vi "OE2012&OE2022_Configure Input Filter.vi"(7 "OE2012&OE2022_\nConfigure Input Filter":T1={"Input Source"=0, "Input Shield Grounding "=0, "Input Coupling "=0, "Input Range"=0, "Signal In Channel"=1} {"Signal In Channel" items=["Signal In 1"=1, "Signal In 2"=2]; "Input Range" items=["5V", "1V", "200mV", "50mV", "10mV", "2mV", "1mV"]; "Input Coupling" items=["AC", "DC"]; "Input Shield Grounding" items=["Float", "Ground"]; "Input Source" items=["A", "A-B", "Current"]}, 8 "Error in (no error)":errorcluster caption="error out（no error）", 9 "Remote Mode":u16(ring) items=["USB", "RS232", "GPIB", "Ethernet"], 10 "Connection ID in":refnum<k5>, 11 "VISA resource name":refnum<visa-resource-name>) -> (0 "Error out":errorcluster caption="error out", 1 "Output String":string, 2 "Connection ID out":refnum<k5>, 3 "VISA resource  out":refnum<visa-resource-name>)   [LabVIEW 2011]
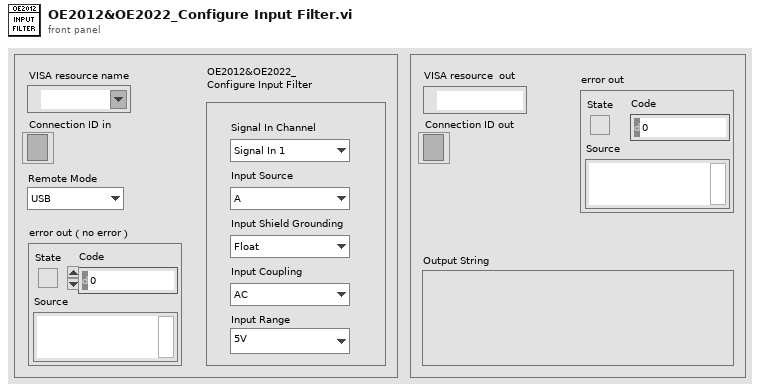
[diagram p1: front panel]
types:
  T1 = cluster{"Input Source":u16, "Input Shield Grounding ":u16, "Input Coupling ":u16, "Input Range":u16, "Signal In Channel":u16}
  T2 = enum16{"ISRC", "IGND", "ICPL", "ILIN", "PHAS", "FMOD", "RSLP", "FREQ", "SWPT", "SLLM", "SULM", "SSLL", "SSLG", "STLM", "SWRM", "IRNG", "SENS", "RMOD", "OFLT", "OFSL", "SYNC", "DMOD", "HARM", "DARB", "SWVT", "SLVL", "SVLL", "SVUL", "SVSL", "SVSG", "SVTM", "SVRM", "RALL", "SNAP", "OUTP", "OAUX", "COUT", "CAUX", "COFP", "CEXP", "FPOP", "OEXP", "*IDN", "*RST", "OVLD", "INOV", "GNOV", "*PLL", "SSET", "RSET", "AGAN", "APHS", "ARSV", "ASCL", "EQCD", "EQCS", "SPED", "SRAT", "SLEN", "SSLE", "STRG", "SPRM", "STRD", "PAUS", "REST", "SPTS", "TRCA", "TEMP", "RSTU", "IHNZ", "DEQU", "SADD", "ARNG", "CSPE", "ISRCD", "IGNDD", "ICPLD", "ILIND", "PHASD", "FMODD", "RSLPD", "FREQD", "SWPTD", "SLLMD", "SULMD", "SSLLD", "SSLGD", "STLMD", "SWRMD", "SENSD", "RMODD", "OFLTD", "OFSLD", "SYNCD", "HARMD", "EQCDD", "EQCSD", "SNAPD", "OUTPD", "SWVTD", "SLVLD", "SVLLD", "SVULD", "SVSLD", "SVSGD", "SVTMD", "SVRMD", "SVDCD", "ARSVD", "AGAND", "APHSD", "ASCLD", "FPOPD", "CAUXD", "OEXPD", "SPEDD", "SRATD", "SLEND", "SSLED", "STRGD", "SPRMD", "STRDD", "PAUSD", "RESTD", "SPTSD", "TRCAD", "*IDND", "*RSTD", "INOVD", "GNOVD", "*PLLD", "SSETD", "RSETD"}
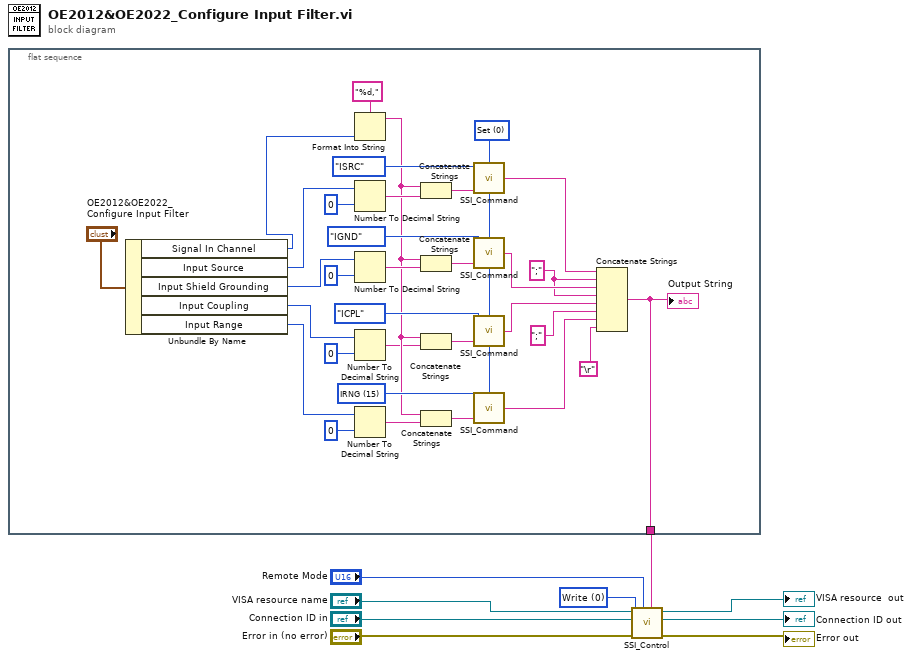
[diagram p0: block diagram]
diagram:
  w7 = u16 0 items=["Write", "Read"] ("Control")
  n1 = flat-sequence {
    tunnel: [w25] -> w1
    frame #0 {
      w24 = u16 15 items=["ISRC", "IGND", "ICPL", "ILIN", "PHAS", "FMOD", "RSLP", "FREQ", "SWPT", "SLLM", "SULM", "SSLL", "SSLG", "STLM", "SWRM", "IRNG", "SENS", "RMOD", "OFLT", "OFSL", "SYNC", "DMOD", "HARM", "DARB", "SWVT", "SLVL", "SVLL", "SVUL", "SVSL", "SVSG", "SVTM", "SVRM", "RALL", "SNAP", "OUTP", "OAUX", "COUT", "CAUX", "COFP", "CEXP", "FPOP", "OEXP", "*IDN", "*RST", "OVLD", "INOV", "GNOV", "*PLL", "SSET", "RSET", "AGAN", "APHS", "ARSV", "ASCL", "EQCD", "EQCS", "SPED", "SRAT", "SLEN", "SSLE", "STRG", "SPRM", "STRD", "PAUS", "RSET", "SPTS", "TRCA", "TEMP", "RSTU", "INHZ", "DEQU", "SADD", "ARNG", "CSPE", "ISRCD", "IGNDD", "ICPLD", "ILIND", "PHASD", "FMODD", "RSLPD", "FREQD", "SWPTD", "SLLMD", "SULMD", "SSLLD", "SSLGD", "STLMD", "SWRMD", "SENSD", "RMODD", "OFLTD", "OFSLD", "SYNCD", "HARMD", "EQCDD", "EQCSD", "SNAPD", "OUTPD", "SWVTD", "SLVLD", "SVLLD", "SVULD", "SVSLD", "SVSGD", "SVTMD", "SVRMD", "SVDCD", "ARSVD", "AGAND", "APHSD", "ASCLD", "FPOPD", "CAUXD", "OEXPD", "SPEDD", "SRATD", "SLEND", "SSLED", "STRGD", "SPRMD", "STRDD", "PAUSD", "RESTD", "SPTSD", "TRCAD", "*IDND", "*RSTD", "INOVD", "GNOVD", "*PLLD", "SSETD", "RSETD", "RALLD"] ("Command Type")
      w26 = ";" ("字符串")
      w21 = u16 0 items=["Set", "Query"] ("Opera")
      n2 = Unbundle By Name("OE2012&OE2022_\nConfigure Input Filter") -> ("Signal In Channel"=w20:u16, "Input Source"=w41:u16, "Input Shield Grounding"=w40:u16, "Input Coupling"=w39:u16, "Input Range"=w38:u16)
      n3 = Format Into String(format string="%d," ("格式字符串"), w20) -> (resulting string=w15:string)  [unwired: 2 in, 1 out]
      n4 = Number To Decimal String(number=w41, width (-)=i16 0 ("精度(6)")) -> (decimal integer string=w18:string)
      n5 = Number To Decimal String(number=w40, width (-)=i16 0 ("精度(6)")) -> (decimal integer string=w16:string)
      n6 = Number To Decimal String(number=w39, width (-)=i16 0 ("精度(6)")) -> (decimal integer string=w13:string)
      n7 = Number To Decimal String(number=w38, width (-)=i16 0 ("精度(6)")) -> (decimal integer string=w14:string)
      n8 = Concatenate Strings(w15, w18) -> (w17:string)
      n9 = Concatenate Strings(w15, w16) -> (w11:string)
      n10 = Concatenate Strings(w15, w13) -> (w12:string)
      n11 = Concatenate Strings(w15, w14) -> (w10:string)
      n12 = call "SSI_Command.vi"("Opera"=w21, "Paramter"=w17, "Command Type"=T2."ISRC") -> ("Output string"=w33:string)  [unwired: 1 in]
      n13 = call "SSI_Command.vi"("Opera"=w21, "Paramter"=w11, "Command Type"=T2."IGND") -> ("Output string"=w32:string)  [unwired: 1 in]
      n14 = call "SSI_Command.vi"("Opera"=w21, "Paramter"=w12, "Command Type"=T2."ICPL") -> ("Output string"=w27:string)  [unwired: 1 in]
      n15 = call "SSI_Command.vi"("Opera"=w21, "Paramter"=w10, "Command Type"=w24) -> ("Output string"=w28:string)  [unwired: 1 in]
      n16 = Concatenate Strings(w33, w26, w32, w26, w27, ";" ("字符串"), w28, "\r") -> (w25:string)
      "Output String" <- w25
    }
  }
  n17 = call "SSI_Control.vi"("Write Buffer"=w1, "Remote Mode"="Remote Mode", "Error in (no error)"="Error in (no error)", "Control"=w7, "Connection ID in"="Connection ID in", "VISA resource name"="VISA resource name") -> ("Error out"=→"Error out":errorcluster, "Connection ID out"=→"Connection ID out":refnum<k5>, "VISA resource  out"=→"VISA resource  out":refnum<visa-resource-name>)  [unwired: 2 in, 1 out]
